vi "CRYGraph Property Window Main.vi"(9 "TabName":string, 10 "pGraph VI In":refnum<vi>) -> ()   [LabVIEW 2013]
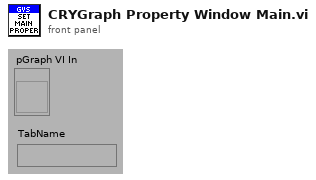
[diagram p1: front panel]
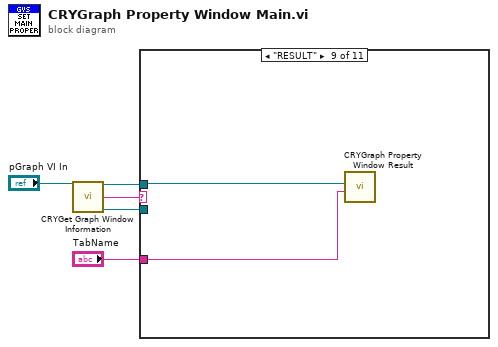
[diagram p0: block diagram]
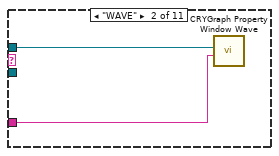
[diagram p3: hidden frame]
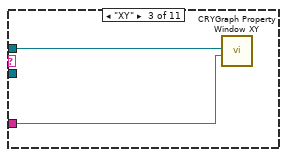
[diagram p4: hidden frame]
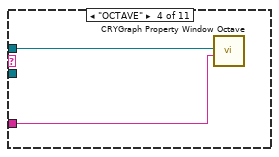
[diagram p5: hidden frame]
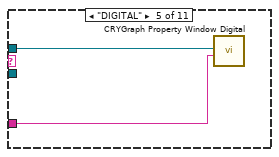
[diagram p6: hidden frame]
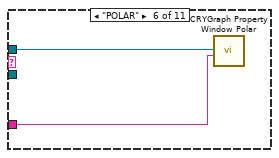
[diagram p7: hidden frame]
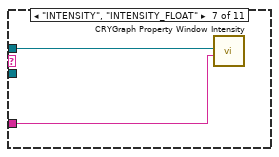
[diagram p8: hidden frame]
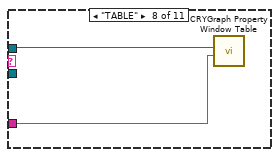
[diagram p9: hidden frame]
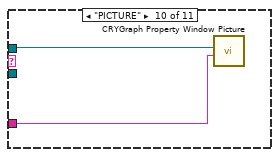
[diagram p10: hidden frame]
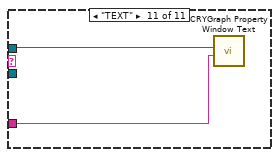
[diagram p11: hidden frame]
diagram:
  n1 = call "CRYGet Graph Window Information.vi"("pGraph VI In"="pGraph VI In") -> ("pGraph VI Out"=w5:refnum<vi>, "Graph Type Out"=w3:string, "Legend Ref Out"=w4:refnum<vi>)  [unwired: 2 in, 10 out]
  n2 = case shown="\"RESULT\"" w3 {
    tunnel: w5 -> [_ w7 w9 w11 w13 w15 w17 w19 w21 w23 w25]
    tunnel: w4 -> [_ _ _ _ _ _ _ _ _ _ _]
    tunnel: "TabName" -> [_ w6 w8 w10 w12 w14 w16 w18 w20 w22 w24]
    frame Default {
    }
    frame "WAVE" {
      n3 = call "CRYGraph Property Window Wave.vi"("Tab Name"=w6, "Graph VI Ref"=w7) -> ()  [unwired: 5 in, 5 out]
    }
    frame "XY" {
      n4 = call "CRYGraph Property Window XY.vi"("TabName"=w8, "Graph VI Ref"=w9) -> ()  [unwired: 5 in, 5 out]
    }
    frame "OCTAVE" {
      n5 = call "CRYGraph Property Window Octave.vi"("TabName"=w10, "Graph VI Ref"=w11) -> ()  [unwired: 4 in, 6 out]
    }
    frame "DIGITAL" {
      n6 = call "CRYGraph Property Window Digital.vi"("Tab Name"=w12, "Graph VI Ref"=w13) -> ()  [unwired: 4 in, 6 out]
    }
    frame "POLAR" {
      n7 = call "CRYGraph Property Window Polar.vi"("TabName"=w14, "Graph VI Ref"=w15) -> ()  [unwired: 10 in]
    }
    frame "INTENSITY", "INTENSITY_FLOAT" {
      n8 = call "CRYGraph Property Window Intensity.vi"("Tab Name"=w16, "Graph VI Ref"=w17) -> ()  [unwired: 10 in]
    }
    frame "TABLE" {
      n9 = call "CRYGraph Property Window Table.vi"("Tab Name"=w18, "Graph VI Ref"=w19) -> ()  [unwired: 9 in]
    }
    frame "RESULT" {
      n10 = call "CRYGraph Property Window Result.vi"("Tab Name"=w20, "Graph VI Ref"=w21) -> ()  [unwired: 9 in]
    }
    frame "PICTURE" {
      n11 = call "CRYGraph Property Window Picture.vi"("Tab Name"=w22, "Graph VI Ref"=w23) -> ()  [unwired: 9 in]
    }
    frame "TEXT" {
      n12 = call "CRYGraph Property Window Text.vi"("Tab Name"=w24, "Graph VI Ref"=w25) -> ()  [unwired: 9 in]
    }
  }
